vi "AddParentAndChild.vi"(9 "Child":refnum<class "Person.lvclass">, 10 "Parent":refnum<class "Person.lvclass">, 11 "Relationships In":refnum<class "Relationships.lvclass">) -> (3 "Relationships Out":refnum<class "Relationships.lvclass">)   [LabVIEW 2018, in "Relationships.lvclass"]
uses:
  Relationships.lvclass
  Person/Person.lvclass
  IRelationshipBrowser/Relationship.ctl
  Relationships.lvclass/Relationships.ctl
  IRelationshipBrowser/IRelationshipBrowser.lvclass
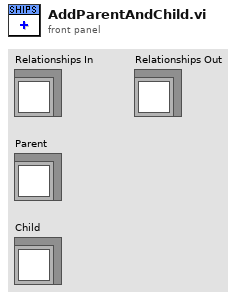
[diagram p1: front panel]
types:
  T1 = typedef "IRelationshipBrowser.lvclass/Relationship.ctl" = enum16{"Sibling", "Child", "Parent"}
  T2 = cluster{"Person A":refnum<class "Person.lvclass">, "Person B":refnum<class "Person.lvclass">, "Relationship A->B":T1}
  T3 = cluster{"Person A":refnum<class "Person.lvclass">, "Person B":refnum<class "Person.lvclass">, "Relationship A->B":T1}[]
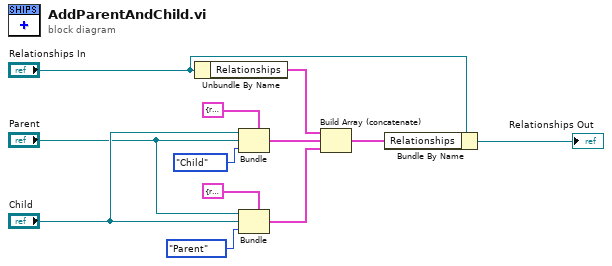
[diagram p0: block diagram]
diagram:
  n1 = Unbundle By Name("Relationships In") -> ("Relationships"=w9:T3)
  n2 = Bundle(cluster=T2 {"Person A"=refnum, "Person B"=refnum, "Relationship A->B"=enum."Sibling"} ("Cluster"), "Person A"="Child", "Person B"="Parent", "Relationship A->B"=Relationship."Child" ("Relationship")) -> (w7:T2)
  n3 = Bundle(cluster=T2 {"Person A"=refnum, "Person B"=refnum, "Relationship A->B"=enum."Sibling"} ("Cluster"), "Person A"="Parent", "Person B"="Child", "Relationship A->B"=Relationship."Parent" ("Relationship")) -> (w2:T2)
  n4 = Build Array (concatenate)(w9, w7, w2) -> (w8:T3)
  n5 = Bundle By Name(cluster="Relationships In", "Relationships"=w8) -> (→"Relationships Out":refnum<class "Relationships.lvclass">)
